vi "Chapter seven main.vi"() -> ()   [LabVIEW 2013]
uses:
  General VIs/Tesla/Control/Command Enum.ctl
  <vilib>/Utility/NIReport.llb/NI_report.lvclass
  <vilib>/regexp/Match Regular Expression.xnode
  <vilib>/Utility/NIReport.llb/Append Report Text (str wrap).vi
panel:
  out "appended path":path
  out "index":i32
  in  "error in":errorcluster
  out "error out":errorcluster
  in  "Tab Control":T1(tab)
  in  "Protocol":bool
  in  "Text Base":bool
  in  "Network":bool
  in  "Commence":bool
  out "IP address":i32
  out "offset past match":i32
  out "concatenated string":string
  out "Ping Cout":i32
  out "VP/F1 5":bool
  out "VP/F1 4":bool
  out "VP/F1 3":bool
  out "VP/F1 2":bool
  out "VP/F1":bool
  out "Hex 5":bool
  out "Hex 4":bool
  out "Hex 3":bool
  out "Hex 2":bool
  out "Hex 1":bool
  out "Percent 5":dbl
  out "Percent 4":dbl
  out "Percent 3":dbl
  out "Percent 2":dbl
  out "Percent 1":dbl
  out "Voltage 5":dbl
  out "Voltage 4":dbl
  out "Voltage 3":dbl
  out "Voltage 2":dbl
  out "Voltage 1":dbl
  out "Pass/Fail1 5":bool
  out "Pass/Fail1 4":bool
  out "Pass/Fail1 3":bool
  out "Pass/Fail1 2":bool
  out "Pass/Fail1":bool
  out "Value in Flpating Point":dbl
  out "Hex String":string
  in  "Path Protocol test":path=path "C:/Users/barddya/Desktop/Tesla_Program/test3.bin"
  in  "Panic Stop":bool=TRUE
  in  "Done press continue":bool
  # "Pass/Fail"
  # "Voltage"
  # "Precent"
  # "Is Hex"
  # "Results"
  # "Response 1"
  # "Response 2"
  # "Response 3"
  # "Response 4"
  # "Response 5"
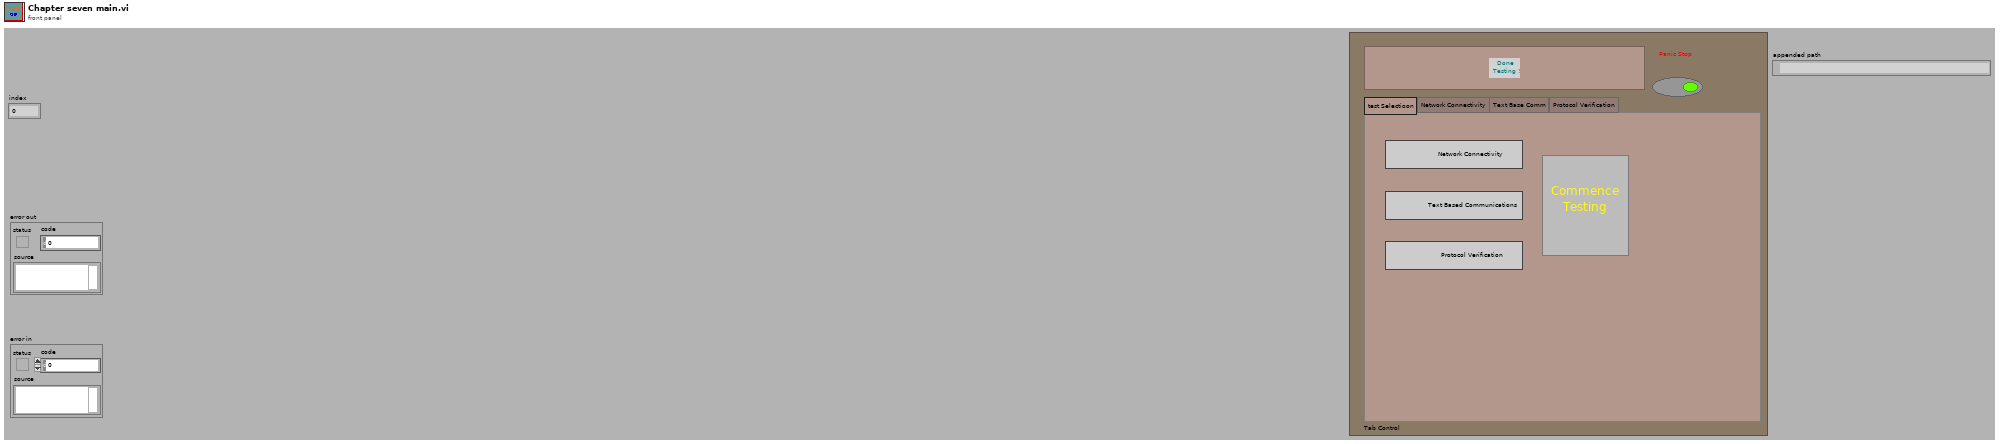
[diagram p1: front panel]
types:
  T1 = enum32{"test Selectioon", "Network Connectivity", "Text Base Comm", "Protocol Verification"}
  T2 = typedef "Command Enum.ctl" = enum16{"Test Selection", "Network", "Text Base", "Protocol", "Restart_Print", "Stop"}
  T3 = enum16{"big-endian, network order", "native, host order", "little-endian"}
  T4 = enum16{"open", "replace", "create", "open or create", "replace or create", "replace or create with confirmation"}
  T5 = cluster{"Charset (-1)":i16, "Weight (-1)":i16, "Name":string, "Size":string}
  T6 = enum16{"Standard Report", "HTML", "Word", "Excel"}
  T7 = enum16{"Left Button", "Center Button", "Right Button", "Window Close"}
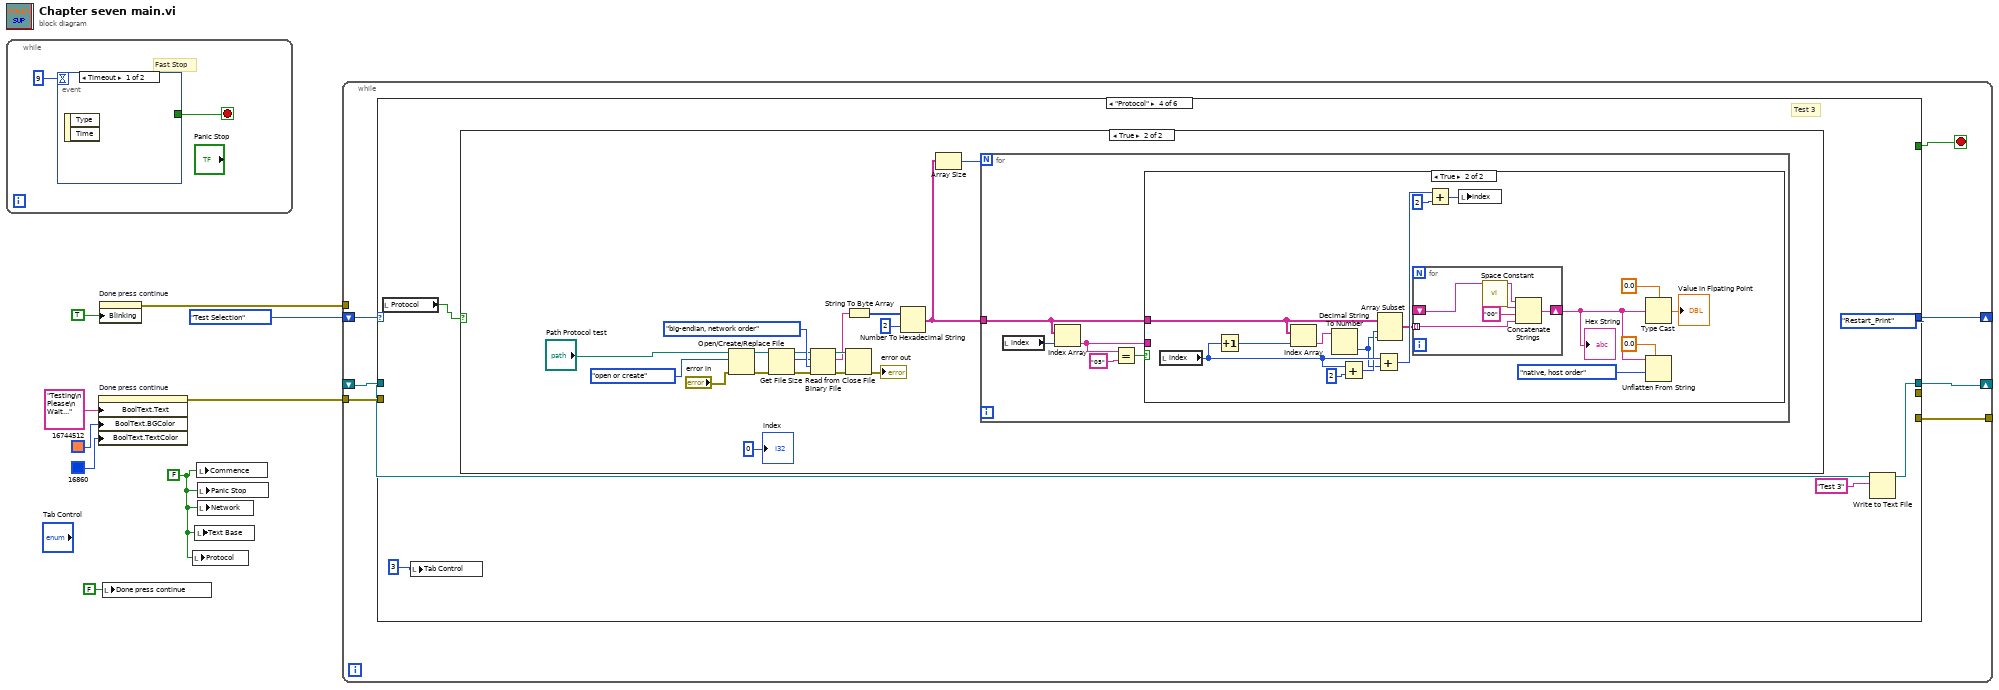
[diagram p0: block diagram]
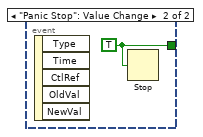
[diagram p2: hidden frame]
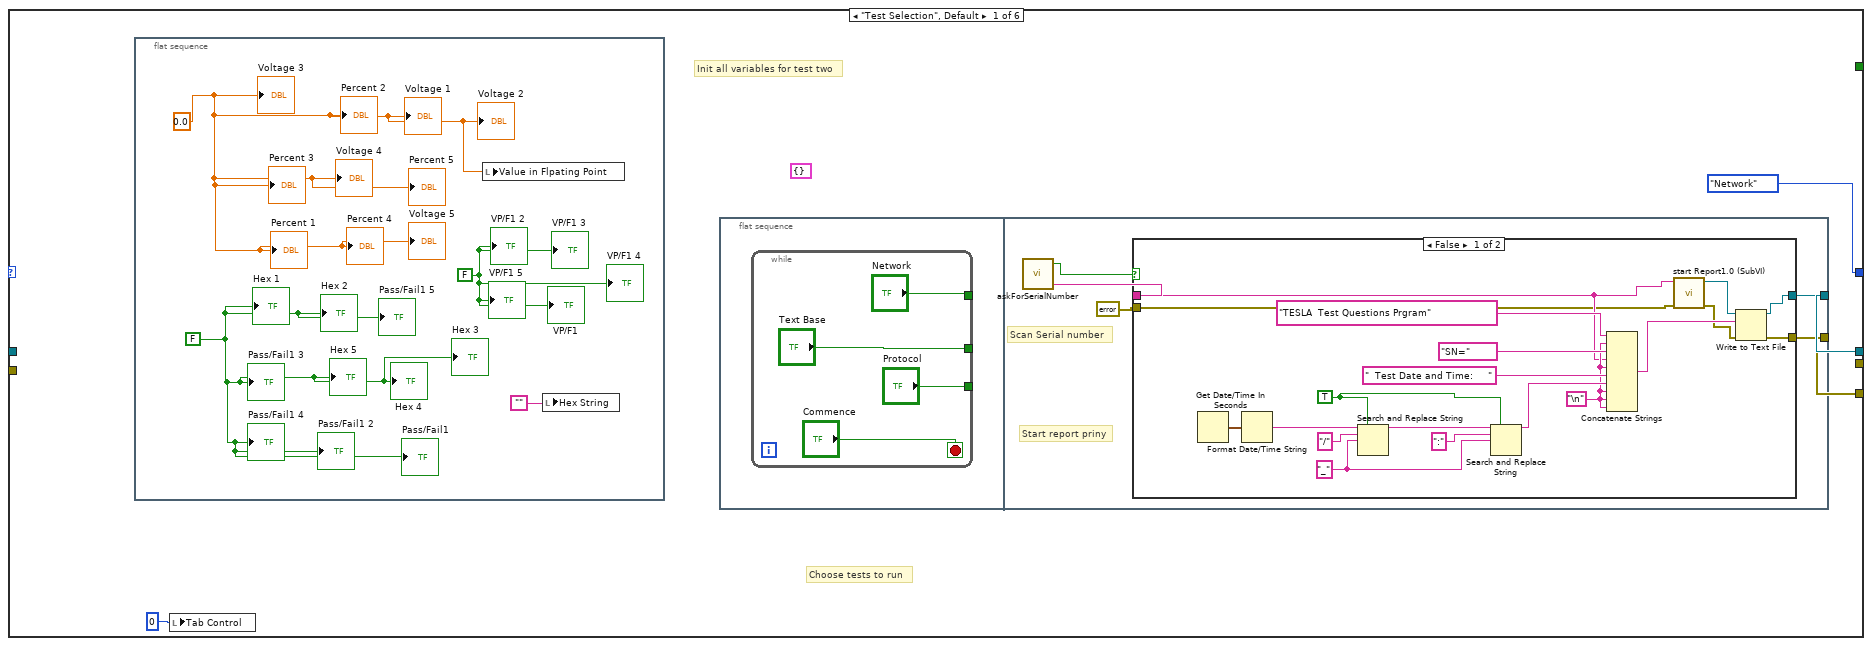
[diagram p3: hidden frame]
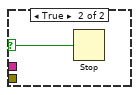
[diagram p4: hidden frame]
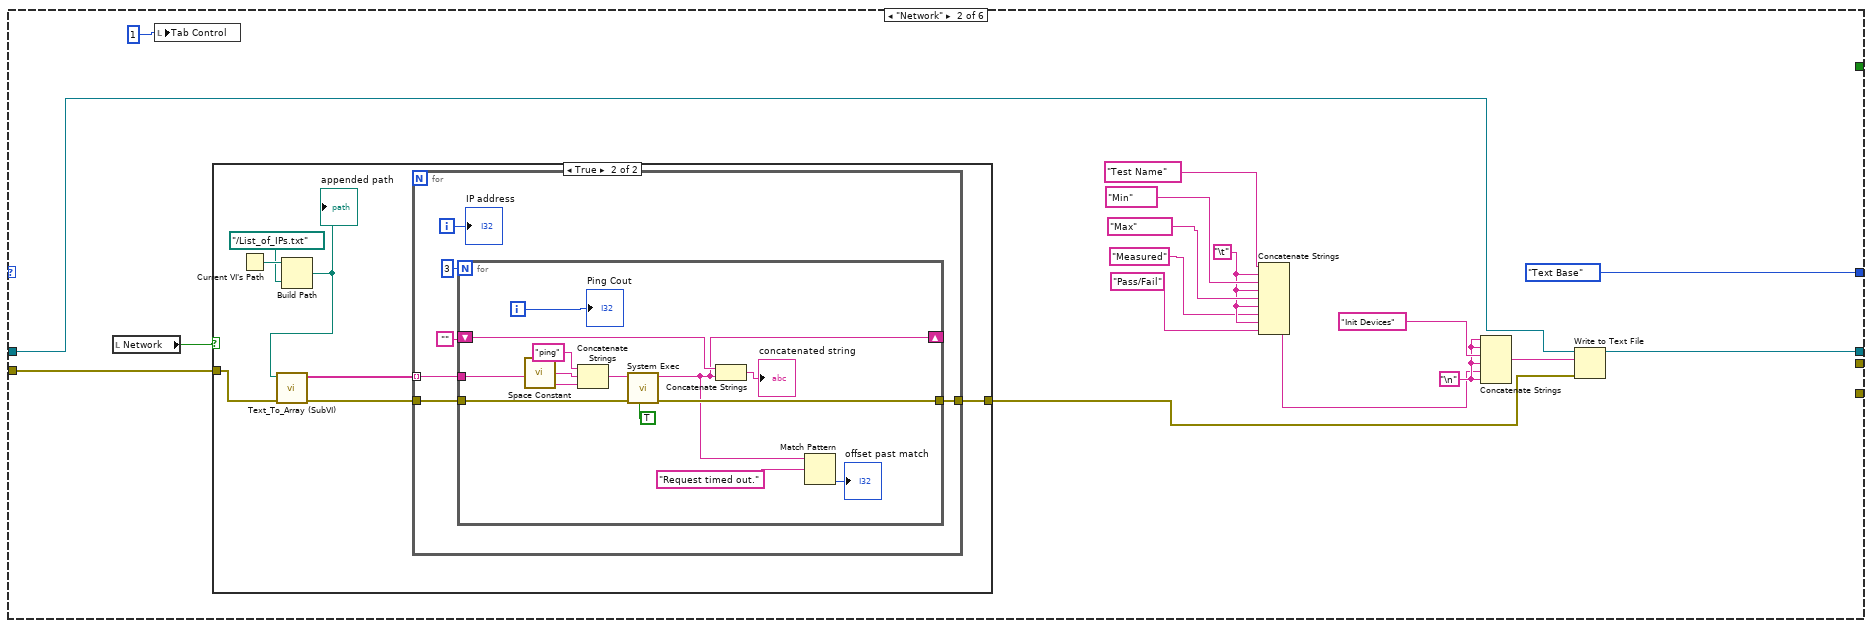
[diagram p5: hidden frame]
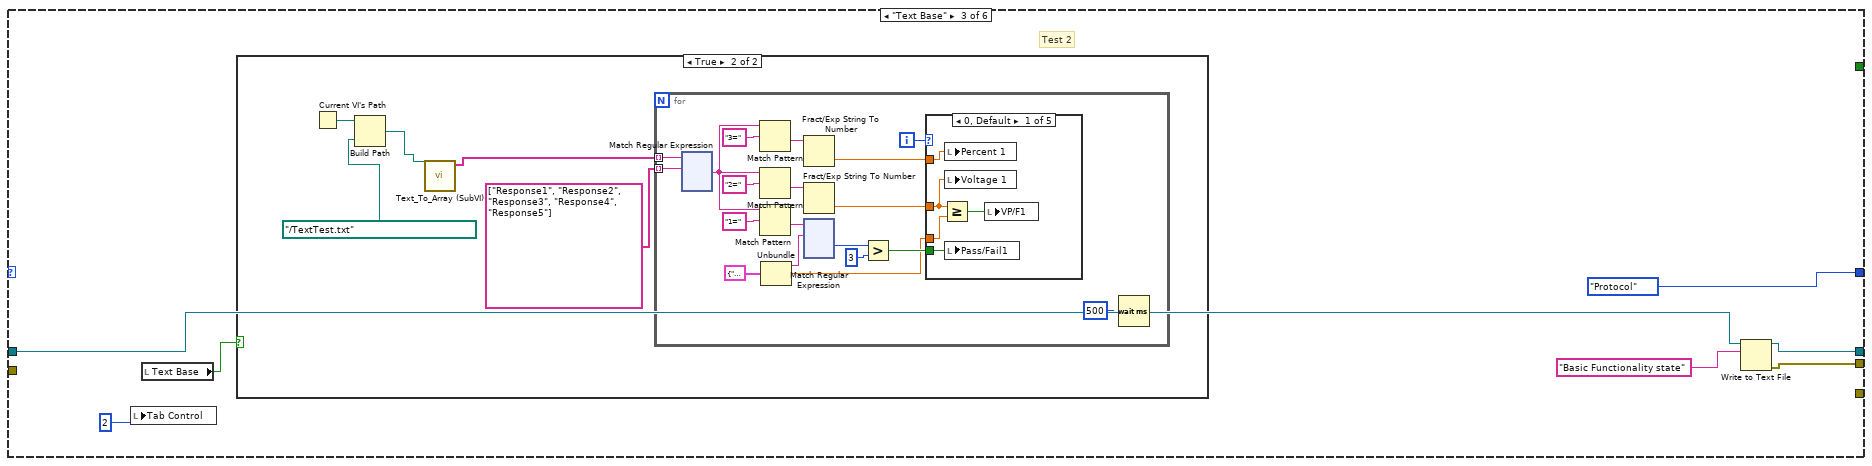
[diagram p7: hidden frame]
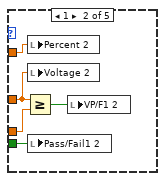
[diagram p9: hidden frame]
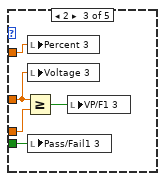
[diagram p10: hidden frame]
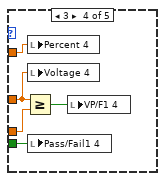
[diagram p11: hidden frame]
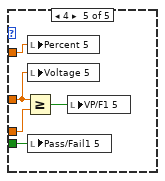
[diagram p12: hidden frame]
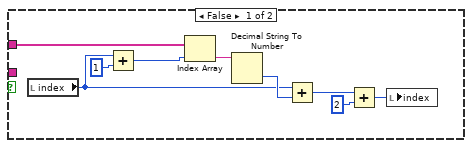
[diagram p14: hidden frame]
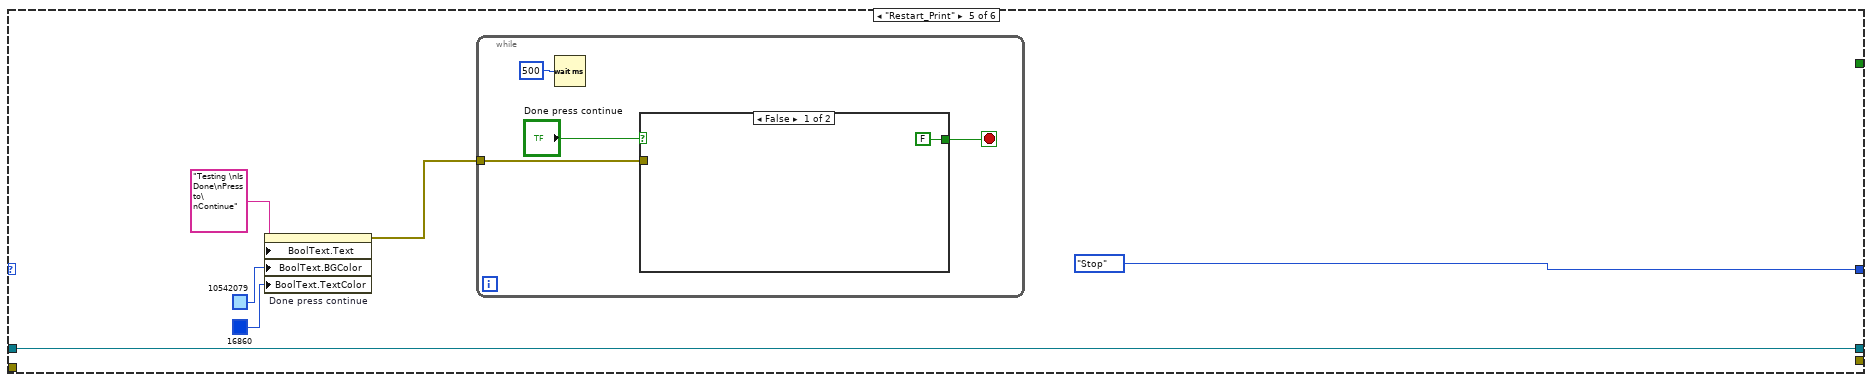
[diagram p15: hidden frame]
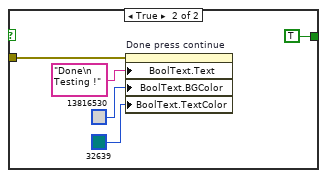
[diagram p16: hidden frame]
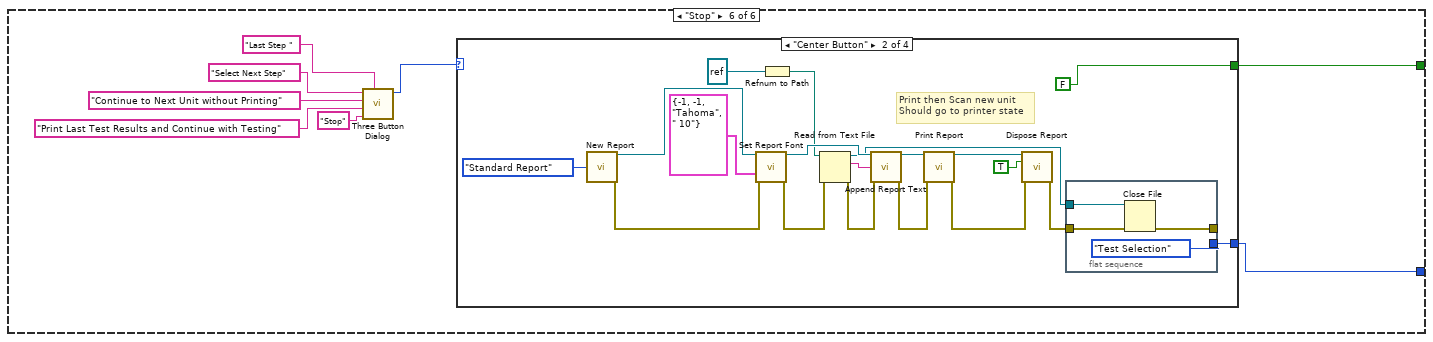
[diagram p17: hidden frame]
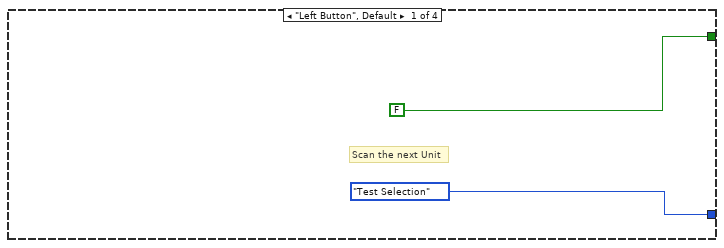
[diagram p18: hidden frame]
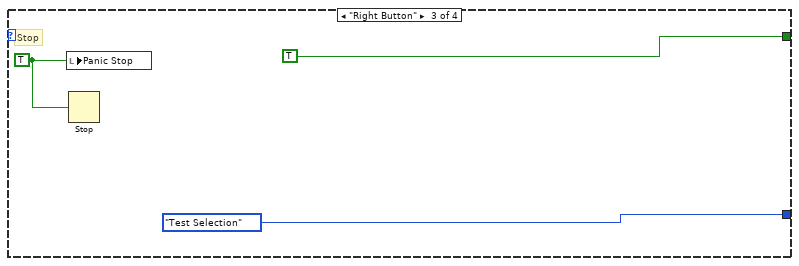
[diagram p19: hidden frame]
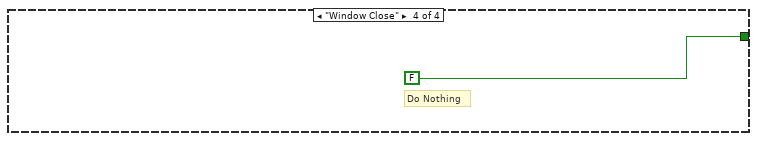
[diagram p20: hidden frame]
diagram:
  w1 = FALSE
  n1 = while {
    stop <- w10 stop-if-true
    # "Fast Stop"
    n2 = event shown="[0] Timeout" {
      selector: _ -> [_ _]
      dyn-events: _ -> [_ _]
      timeout: 9 -> [_ _]
      tunnel: [_ w12] -> w10
      event Timeout {
        n3 = event-data() -> ()  [unwired: 1 in, 2 out]
      }
      event "Panic Stop": Value Change {
        w12 = TRUE
        n4 = event-data() -> ()  [unwired: 1 in, 5 out]
        n5 = Stop(stop? (T)=w12) -> ()
      }
    }
  }
  n6 = property on="Done press continue" class="Bool (strict)"("BoolText.Text"="Testing\n Please\n Wait...", "BoolText.BGColor"=u32 16744512, "BoolText.TextColor"=u32 16860) -> (error out=w7:errorcluster)  [unwired: 2 in, 1 out]
  n7 = property on="Done press continue" class="Bool (strict)"("Blinking"=TRUE) -> (error out=w3:errorcluster)  [unwired: 2 in, 1 out]
  n8 = local write "Done press continue"(FALSE) -> ()
  n9 = local write "Protocol"(w1) -> ()
  n10 = local write "Text Base"(w1) -> ()
  n11 = local write "Commence"(w1) -> ()
  n12 = local write "Panic Stop"(w1) -> ()
  n13 = local write "Network"(w1) -> ()
  n14 = while {
    shift-right: [w18] -> _
    shift-left: Command_Enum."Test Selection" ("Command Enum") -> [w19]
    tunnel: w7 -> [w16]
    tunnel: w3 -> [_]
    shift-right: [w15] -> _
    shift-left: _ -> [w14]
    tunnel: [w13] -> _
    stop <- w17 stop-if-true
    n15 = case shown="\"Protocol\"" w19 {
      tunnel: [Command_Enum."Network" ("Command Enum") Command_Enum."Text Base" ("Command Enum") Command_Enum."Protocol" ("Command Enum") Command_Enum."Restart_Print" ("Command Enum") Command_Enum."Stop" ("Command Enum") w461] -> w18
      tunnel: [_ _ _ _ _ w460] -> w17
      tunnel: w16 -> [_ w67 _ _ _ _]
      tunnel: [w22 w71 w105 w389 w444 _] -> w15
      tunnel: w14 -> [_ w70 w104 w387 w444 _]
      tunnel: [_ _ w106 _ _ _] -> _
      tunnel: [w20 _ _ _ _ _] -> w13
      frame "Test Selection", Default {
        (unwired) cluster{} {}
        # "Choose tests to run"
        # "Init all variables for test two"
        n16 = flat-sequence {
          frame #0 {
            w26 = FALSE
            w27 = FALSE
            w25 = 0.0
            n17 = local write "Value in Flpating Point"(w25) -> ()
            n18 = local write "Hex String"("") -> ()
            "Voltage 5" <- w25
            "Percent 5" <- w25
            "Voltage 3" <- w25
            "Voltage 4" <- w25
            "Voltage 2" <- w25
            "Percent 4" <- w25
            "Percent 3" <- w25
            "Voltage 1" <- w25
            "Percent 2" <- w25
            "Percent 1" <- w25
            "Pass/Fail1 5" <- w27
            "Hex 5" <- w27
            "Pass/Fail1 3" <- w27
            "Pass/Fail1 4" <- w27
            "Pass/Fail1" <- w27
            "Hex 3" <- w27
            "Hex 4" <- w27
            "Hex 2" <- w27
            "Hex 1" <- w27
            "Pass/Fail1 2" <- w27
            "VP/F1 3" <- w26
            "VP/F1 4" <- w26
            "VP/F1 2" <- w26
            "VP/F1" <- w26
            "VP/F1 5" <- w26
          }
        }
        n19 = local write "Tab Control"(0) -> ()
        n20 = flat-sequence {
          tunnel: [w34] -> w22
          tunnel: [w33] -> w20
          frame #0 {
            n21 = while {
              tunnel: ["Network"] -> _
              tunnel: ["Protocol"] -> _
              tunnel: ["Text Base"] -> _
              stop <- "Commence" stop-if-true
            }
          }
          frame #1 {
            # "Start report priny"
            # "Scan Serial number"
            n22 = call "askForSerialNumber.vi"() -> ("Stop"=w36:bool, "Serial Number scanned"=w35:string)  [unwired: 1 in, 1 out]
            n23 = case shown="False" w36 {
              selector: w36 -> [_ w56]
              tunnel: w35 -> [w40 _]
              tunnel: [w43 _] -> w34
              tunnel: [w41 _] -> w33
              tunnel: errorcluster {"status"=FALSE, "code"=0, "source"=""} ("error constant") -> [w39 _]
              frame False {
                w44 = "\n"
                w53 = TRUE ("replace all? (F)")
                w52 = "_"
                n24 = Get Date/Time In Seconds() -> (seconds since 1Jan1904=w47:timestamp)
                n25 = Format Date/Time String(seconds (now)=w47) -> (date/time string=w48:string)  [unwired: 2 in]
                n26 = Search and Replace String(replace all?=w53, input string=w48, search string="/", replace string=w52) -> (result string=w50:string)  [unwired: 4 in, 3 out]
                n27 = Search and Replace String(replace all?=w53, input string=w50, search string=":", replace string=w52) -> (result string=w55:string)  [unwired: 4 in, 3 out]
                n28 = Concatenate Strings("TESLA  Test Questions Prgram", w44, "SN=", w40, w44, "  Test Date and Time:     ", w55, w44, w44, w44) -> (w42:string)
                n29 = call "start Report1.0 (SubVI).vi"("error in (no error)"=w39, "Serial Number"=w40) -> ("error out"=w38:errorcluster, "Byte Stream File out"=w37:refnum<file>)  [unwired: 8 in]
                n30 = Write to Text File(file (use dialog)=w37, text=w42, error in=w38) -> (refnum out=w43:refnum<file>, error out=w41:errorcluster)  [unwired: 1 in, 1 out]
              }
              frame True {
                n31 = Stop(stop? (T)=w56) -> ()
              }
            }
          }
        }
      }
      frame "Network" {
        w61 = "\t"
        w68 = "\n"
        n32 = local read "Network"() -> (w57:bool)
        n33 = local write "Tab Control"(1) -> ()
        n34 = case shown="True" w57 {
          tunnel: w67 -> [w74 w79]
          tunnel: [w74 w78] -> w66
          frame False {
          }
          frame True {
            n35 = Current VI's Path() -> (path=w77:path)
            n36 = Build Path(base path=w77, name or relative path=path "../List_of_IPs.txt") -> (appended path=w75:path)
            "appended path" <- w75
            n37 = call "Text_To_Array (SubVI).vi"("error in (no error)"=w79, "Path"=w75) -> ("error out"=w80:errorcluster, "Array"=w81:string[])  [unwired: 7 in, 1 out]
            n38 = for {
              tunnel: w81 -> [w85] mode=indexing
              tunnel: w80 -> [w87]
              tunnel: [w86] -> w78
              i -> [w83]
              n39 = for {
                N: 3 -> [_]
                tunnel: w87 -> [w100]
                tunnel: [w99] -> w86
                tunnel: w85 -> [w97]
                shift-right: [w90] -> _
                shift-left: "" -> [w92]
                i -> [w93]
                n40 = call <vilib>:"Space Constant.vi"() -> ("String"=w95:string)
                n41 = Concatenate Strings("ping", w95, w97) -> (w98:string)
                n42 = call <vilib>:"System Exec.vi"("run minimized? (F)"=TRUE, "error in (no error)"=w100, "command line"=w98) -> ("error out"=w99:errorcluster, "standard output"=w90:string)  [unwired: 5 in, 2 out]
                n43 = Concatenate Strings(w92, w90) -> (→"concatenated string":string)
                n44 = Match Pattern(string=w90, regular expression="Request timed out." ("search string/char (-)")) -> (offset past match=→"offset past match":i32)  [unwired: 1 in, 3 out]
                "Ping Cout" <- w93
              }
              "IP address" <- w83
            }
          }
        }
        n45 = Concatenate Strings("Test Name", w61, "Min", w61, "Max", w61, "Measured", w61, "Pass/Fail") -> (w58:string)
        n46 = Concatenate Strings(w68, w68, "Init Devices", w68, w58, w68) -> (w72:string)
        n47 = Write to Text File(file (use dialog)=w70, text=w72, error in=w66) -> (refnum out=w71:refnum<file>)  [unwired: 1 in, 2 out]
      }
      frame "Text Base" {
        # "Test 2"
        n48 = local write "Tab Control"(2) -> ()
        n49 = local read "Text Base"() -> (w102:bool)
        n50 = case shown="True" w102 {
          frame False {
          }
          frame True {
            n51 = Current VI's Path() -> (path=w110:path)
            n52 = Build Path(base path=w110, name or relative path=path "../TextTest.txt") -> (appended path=w108:path)
            n53 = call "Text_To_Array (SubVI).vi"("Path"=w108) -> ("Array"=w111:string[])  [unwired: 8 in, 2 out]
            n54 = for {
              tunnel: w111 -> [w120] mode=indexing
              tunnel: string[] ["Response1", "Response2", "Response3", "Response4", "Response5"] -> [w119] mode=indexing
              i -> [w118]
              n55 = xnode "Match Regular Expression"("input string"=w120, "regular expression"=w119) -> ("after match"=w115:string)  [unwired: 4 in, 4 out]
              n56 = Match Pattern(string=w115, regular expression="3=") -> (after substring=w114:string)  [unwired: 1 in, 3 out]
              n57 = Match Pattern(string=w115, regular expression="2=") -> (after substring=w122:string)  [unwired: 1 in, 3 out]
              n58 = Match Pattern(string=w115, regular expression="1=") -> (after substring=w127:string)  [unwired: 1 in, 3 out]
              n59 = Unbundle(cluster{string, dbl, i32} {"PASS", 3.3, 80}) -> (w130:string, w117:dbl)  [unwired: 1 out]
              n60 = Fract/Exp String To Number(string=w114) -> (number=w113:dbl)  [unwired: 3 in, 1 out]
              n61 = Fract/Exp String To Number(string=w122) -> (number=w121:dbl)  [unwired: 3 in, 1 out]
              n62 = xnode "Match Regular Expression"("input string"=w127, "regular expression"=w130) -> ("offset past match"=w126:i32)  [unwired: 4 in, 4 out]
              n63 = Greater?(x=w126, y=3) -> (0:w124:bool)
              n64 = case shown="0, Default" w118 {
                tunnel: w124 -> [w136 w141 w146 w151 w156]
                tunnel: w121 -> [w135 w140 w145 w150 w155]
                tunnel: w117 -> [w134 w139 w144 w149 w154]
                tunnel: w113 -> [w132 w137 w142 w147 w152]
                frame 0, Default {
                  n65 = Greater Or Equal?(x=w135, y=w134) -> (x >= y?=w133:bool)
                  n66 = local write "Percent 1"(w132) -> ()
                  n67 = local write "Voltage 1"(w135) -> ()
                  n68 = local write "Pass/Fail1"(w136) -> ()
                  n69 = local write "VP/F1"(w133) -> ()
                }
                frame 1 {
                  n70 = Greater Or Equal?(x=w140, y=w139) -> (x >= y?=w138:bool)
                  n71 = local write "Percent 2"(w137) -> ()
                  n72 = local write "Voltage 2"(w140) -> ()
                  n73 = local write "Pass/Fail1 2"(w141) -> ()
                  n74 = local write "VP/F1 2"(w138) -> ()
                }
                frame 2 {
                  n75 = Greater Or Equal?(x=w145, y=w144) -> (x >= y?=w143:bool)
                  n76 = local write "Percent 3"(w142) -> ()
                  n77 = local write "Voltage 3"(w145) -> ()
                  n78 = local write "Pass/Fail1 3"(w146) -> ()
                  n79 = local write "VP/F1 3"(w143) -> ()
                }
                frame 3 {
                  n80 = Greater Or Equal?(x=w150, y=w149) -> (x >= y?=w148:bool)
                  n81 = local write "Percent 4"(w147) -> ()
                  n82 = local write "Voltage 4"(w150) -> ()
                  n83 = local write "Pass/Fail1 4"(w151) -> ()
                  n84 = local write "VP/F1 4"(w148) -> ()
                }
                frame 4 {
                  n85 = Greater Or Equal?(x=w155, y=w154) -> (x >= y?=w153:bool)
                  n86 = local write "Percent 5"(w152) -> ()
                  n87 = local write "Voltage 5"(w155) -> ()
                  n88 = local write "Pass/Fail1 5"(w156) -> ()
                  n89 = local write "VP/F1 5"(w153) -> ()
                }
              }
              n90 = Wait (ms)(milliseconds to wait=500) -> ()  [unwired: 1 out]
            }
          }
        }
        n91 = Write to Text File(file (use dialog)=w104, text="Basic Functionality state") -> (refnum out=w105:refnum<file>, error out=w106:errorcluster)  [unwired: 2 in, 1 out]
      }
      frame "Protocol" {
        # "Test 3"
        n92 = local read "Protocol"() -> (w386:bool)
        n93 = local write "Tab Control"(3) -> ()
        n94 = case shown="True" w386 {
          frame False {
          }
          frame True {
            n95 = Open/Create/Replace File(file path (use dialog)="Path Protocol test", error in="error in", operation (0:open)=T4."open or create") -> (refnum out=w401:refnum<file>, error out=w399:errorcluster)  [unwired: 3 in, 1 out]
            n96 = Get File Size(file=w401, error in=w399) -> (refnum out=w400:refnum<file>, size (in bytes)=w397:i64, 0:w398:errorcluster)
            n97 = Read from Binary File(8:w398, 9:T3."big-endian, network order" ("byte order (0:big-endian, network order)"), 10:w397, 11:w400) -> (0:w404:errorcluster, 2:w396:string, 3:w402:refnum<file>)  [unwired: 2 in, 1 out]
            n98 = String To Byte Array(string=w396) -> (unsigned byte array=w395:u8[])
            n99 = Close File(refnum=w402, error in=w404) -> (error out=→"error out":errorcluster)  [unwired: 1 out]
            n100 = Number To Hexadecimal String(1:2, 2:w395) -> (0:w393:string[])
            n101 = Array Size(array=w393) -> (size(s)=w391:i32)
            n102 = for {
              N: w391 -> [_]
              tunnel: w393 -> [w411]
              n103 = local read "index"() -> (w409:i32)
              n104 = Index Array(array=w411, index=w409) -> (element=w410:string)
              n105 = Equal?(x=w410, y="05") -> (x = y?=w412:bool)
              n106 = case shown="True" w412 {
                tunnel: w411 -> [w420 w435]
                tunnel: w410 -> [_ _]
                frame False {
                  n107 = local read "index"() -> (w417:i32)
                  n108 = Add(x=w417, y=1) -> (x+y=w418:i32)
                  n109 = Index Array(array=w420, index=w418) -> (element=w422:string)
                  n110 = Decimal String To Number(string=w422) -> (number=w421:i32)  [unwired: 2 in, 1 out]
                  n111 = Add(x=w417, y=w421) -> (x+y=w416:i32)
                  n112 = Add(x=w416, y=2) -> (x+y=w414:i32)
                  n113 = local write "index"(w414) -> ()
                }
                frame True {
                  n114 = local read "index"() -> (w433:i32)
                  n115 = Increment(x=w433) -> (x+1=w438:i32)
                  n116 = Index Array(array=w435, index=w438) -> (element=w436:string)
                  n117 = Decimal String To Number(string=w436) -> (number=w429:i32)  [unwired: 2 in, 1 out]
                  n118 = Add(x=w433, y=2) -> (x+y=w431:i32)
                  n119 = Add(x=w433, y=w429) -> (x+y=w434:i32)
                  n120 = Array Subset(array=w435, index=w431, length=w429) -> (w428:string[])
                  n121 = for {
                    tunnel: w428 -> [w442] mode=indexing
                    shift-right: [w443] -> w424
                    shift-left: _ -> [w441]
                    n122 = call <vilib>:"Space Constant.vi"() -> ("String"=w439:string)
                    n123 = Concatenate Strings(w441, w439, "00", w442) -> (w443:string)
                  }
                  "Hex String" <- w424
                  n124 = Add(x=w434, y=2) -> (x+y=w430:i32)
                  n125 = local write "index"(w430) -> ()
                  n126 = Type Cast(type=0.0, x=w424) -> (*(type *) &x=→"Value in Flpating Point":dbl)
                  n127 = Unflatten From String(type=0.0, binary string=w424, byte order (0:big-endian, network order)=T3."native, host order") -> ()  [unwired: 2 in, 3 out]
                }
              }
            }
            "index" <- 0
          }
        }
        n128 = Write to Text File(file (use dialog)=w387, text="Test 3") -> (refnum out=w389:refnum<file>)  [unwired: 2 in, 2 out]
      }
      frame "Restart_Print" {
        n129 = property on="Done press continue" class="Bool (strict)"("BoolText.Text"="Testing \nIs Done\nPress to\nContinue", "BoolText.BGColor"=u32 10542079, "BoolText.TextColor"=u32 16860) -> (error out=w448:errorcluster)  [unwired: 2 in, 1 out]
        n130 = while {
          tunnel: w448 -> [w451]
          stop <- w450 stop-if-true
          n131 = Wait (ms)(milliseconds to wait=500) -> ()  [unwired: 1 out]
          n132 = case shown="False" "Done press continue" {
            tunnel: [FALSE TRUE] -> w450
            tunnel: w451 -> [_ w456]
            frame False {
            }
            frame True {
              n133 = property on="Done press continue" class="Bool (strict)"(error in=w456, "BoolText.Text"="Done\n Testing !", "BoolText.BGColor"=u32 13816530, "BoolText.TextColor"=u32 32639) -> ()  [unwired: 1 in, 2 out]
            }
          }
        }
      }
      frame "Stop" {
        n134 = call <vilib>:"Three Button Dialog.vi"("Window Title (\"\")"="Last Step " ("Window Title (\"\")"), "Right Button Text (\"Cancel\")"="Stop" ("Window Title (\"\")"), "Center Button Text (\"No\")"="Print Last Test Results and Continue with Testing" ("Window Title (\"\")"), "Left Button Text (\"Yes\")"="Continue to Next Unit without Printing" ("Window Title (\"\")"), "message"="Select Next Step" ("Window Title (\"\")")) -> ("Which Button?"=w467:T7)  [unwired: 6 in]
        n135 = case shown="\"Center Button\"" w467 {
          tunnel: [Command_Enum."Test Selection" ("Command Enum") w472 Command_Enum."Test Selection" ("Command Enum") _] -> w461
          tunnel: [FALSE FALSE TRUE FALSE] -> w460
          frame "Left Button", Default {
            # "Scan the next Unit"
          }
          frame "Center Button" {
            # "Print then Scan new unit\nShould go to printer state"
            n136 = call <vilib>:"New Report.vi"("report type"=T6."Standard Report") -> ("report out"=w485:refnum<class "NI_report.lvclass">, "error out"=w486:errorcluster)  [unwired: 13 in]
            n137 = call-dynamic "Set Report Font.vi"("report in"=w485, "font settings"=T5 {"Charset (-1)"=-1, "Weight (-1)"=-1, "Name"="Tahoma", "Size"=" 10"}, "error in (no error)"=w486) -> ("report out"=w484:refnum<class "NI_report.lvclass">, "error out"=w483:errorcluster)  [unwired: 10 in, 1 out]
            n138 = Refnum to Path(1:refnum<file> refnum ("refnum")) -> (0:w471:path)
            n139 = Read from Text File(file (use dialog)=w471, error in=w483) -> (refnum out=w473:refnum<file>, text=w482:string, error out=w481:errorcluster)  [unwired: 2 in, 1 out]
            n140 = call-poly <vilib>:"Append Report Text.vi"("report in"=w484, "text"=w482, "error in (no error)"=w481) -> ("report out"=w480:refnum<class "NI_report.lvclass">, "error out"=w477:errorcluster)  [unwired: 9 in, 2 out]
            n141 = call-dynamic "Print Report.vi"("report in"=w480, "error in (no error)"=w477) -> ("report out"=w478:refnum<class "NI_report.lvclass">, "error out"=w479:errorcluster)  [unwired: 12 in]
            n142 = call-dynamic "Dispose Report.vi"("report in"=w478, "wait until printing completed? (T)"=TRUE, "error in (no error)"=w479) -> ("error out"=w474:errorcluster)  [unwired: 12 in]
            n143 = flat-sequence {
              tunnel: w474 -> [w492]
              tunnel: [w491] -> _
              tunnel: w473 -> [w490]
              tunnel: [Command_Enum."Test Selection" ("Command Enum")] -> w472
              frame #0 {
                n144 = Close File(refnum=w490, error in=w492) -> (error out=w491:errorcluster)  [unwired: 1 out]
              }
            }
          }
          frame "Right Button" {
            w493 = TRUE
            # "Stop"
            n145 = local write "Panic Stop"(w493) -> ()
            n146 = Stop(stop? (T)=w493) -> ()
          }
          frame "Window Close" {
            # "Do Nothing"
          }
        }
      }
    }
  }
